vi "Insert Error.vi"(8 "error in":errorcluster, 10 "err":errorcluster, 11 "Instrument in":refnum<class "Instrument.lvclass">) -> (0 "error out":errorcluster, 2 "error?":bool, 3 "Instrument out":refnum<class "Instrument.lvclass">)   [LabVIEW 2018, in "Instrument.lvclass"]
doc: "Insert an error into the error queue in the Instrument class. If the queue has been recently cleared (as indicated by the Error to Handle? flag set to false, then set this flag so that errors may be properly handled."
uses:
  Instrument.lvclass
  Instrument.lvclass/Instrument.ctl
  state.ctl
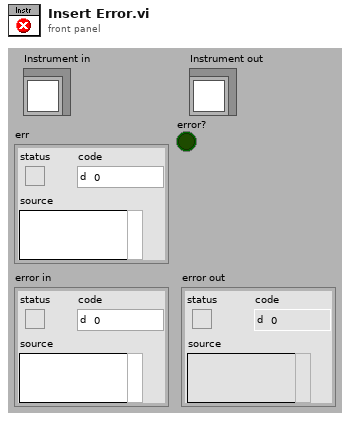
[diagram p1: front panel]
types:
  T1 = typedef "Instrument.lvclass/state.ctl" = enum8{"Configure", "Acquire", "Wait", "Quit", "Handle Error", "NOOP"}
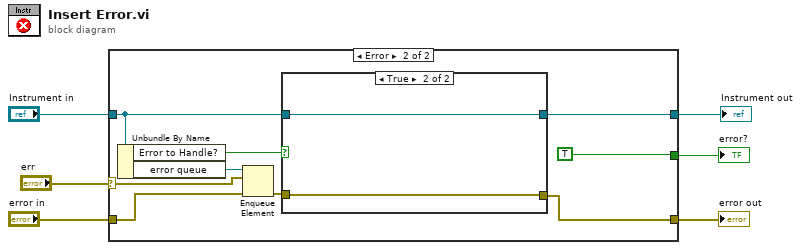
[diagram p0: block diagram]
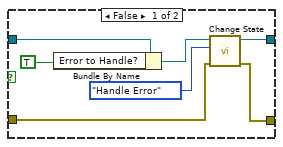
[diagram p3: hidden frame]
diagram:
  n1 = case shown="Error" "err" {
    selector: "err" -> [_ w15]
    tunnel: "Instrument in" -> [w7 w13]
    tunnel: "error in" -> [w8 w16]
    tunnel: [w8 w10] -> w5
    tunnel: [_ TRUE] -> w1
    tunnel: [w7 w9] -> w3
    frame No Error {
    }
    frame Error {
      n2 = Unbundle By Name(w13) -> ("Error to Handle?"=w12:bool, "error queue"=w17:refnum<queue>)
      n3 = Enqueue Element(queue=w17, element=w15, error in (no error)=w16) -> (error out=w11:errorcluster)  [unwired: 1 in, 2 out]
      n4 = case shown="True" w12 {
        tunnel: w13 -> [w23 w25]
        tunnel: [w21 w25] -> w9
        tunnel: w11 -> [w19 w26]
        tunnel: [w18 w26] -> w10
        frame False {
          n5 = Bundle By Name(cluster=w23, "Error to Handle?"=TRUE) -> (w22:refnum<class "Instrument.lvclass">)
          n6 = call "Change State.vi"("error in"=w19, "instr state"=state."Handle Error", "Instrument in"=w22) -> ("error out"=w18:errorcluster, "Instrument out"=w21:refnum<class "Instrument.lvclass">)  [unwired: 7 in]
        }
        frame True {
        }
      }
    }
  }
  "error out" <- w5
  "Instrument out" <- w3
  "error?" <- w1
